vi "buildRampUpWaveform.vi"(4 "Fs":dbl=10000.0, 6 "square wave duty cycle (%)":dbl=20.0 format="%0.2f", 7 "signal type":T1(ring)=enum."Square Wave", 8 "input cluster":cluster{"Fs":dbl, "#s":dbl}={"Fs"=1000.0, "#s"=1000.0}, 9 "amplitude":dbl=2.5, 10 "freq":dbl=40.0, 11 "sec rampup":dbl=0.5 format="%#_13g") -> (3 "rampUp out":waveform(dbl)={"t0"=timestamp(0 s since 1904-01-01), "dt"=1.0, "Y"=array[62500 elements]})   [LabVIEW 2018]
uses:
  <vilib>/Waveform/WDTOps.llb/WDT Append Waveforms DBL.vi
  <vilib>/measure/NI_MABase.lvlib
panel:
  out "output cluster":cluster{"Fs":dbl, "#s":dbl}
  out "N":i32
  out "Waveform Graph":waveform(dbl)(graph)={"t0"=timestamp(0 s since 1904-01-01), "dt"=1.0, "Y"=[]} caption="Optostim waveform"
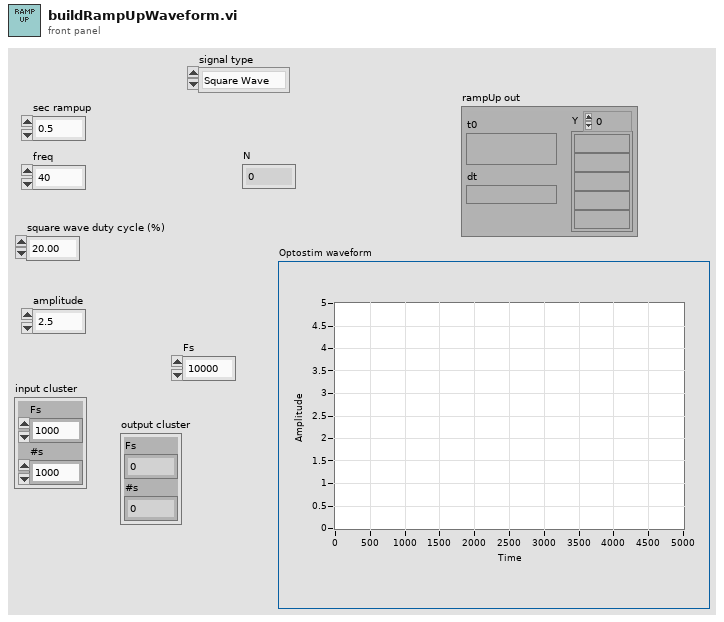
[diagram p1: front panel]
types:
  T1 = enum16{"Sine Wave", "Triangle Wave", "Square Wave", "Sawtooth Wave"}
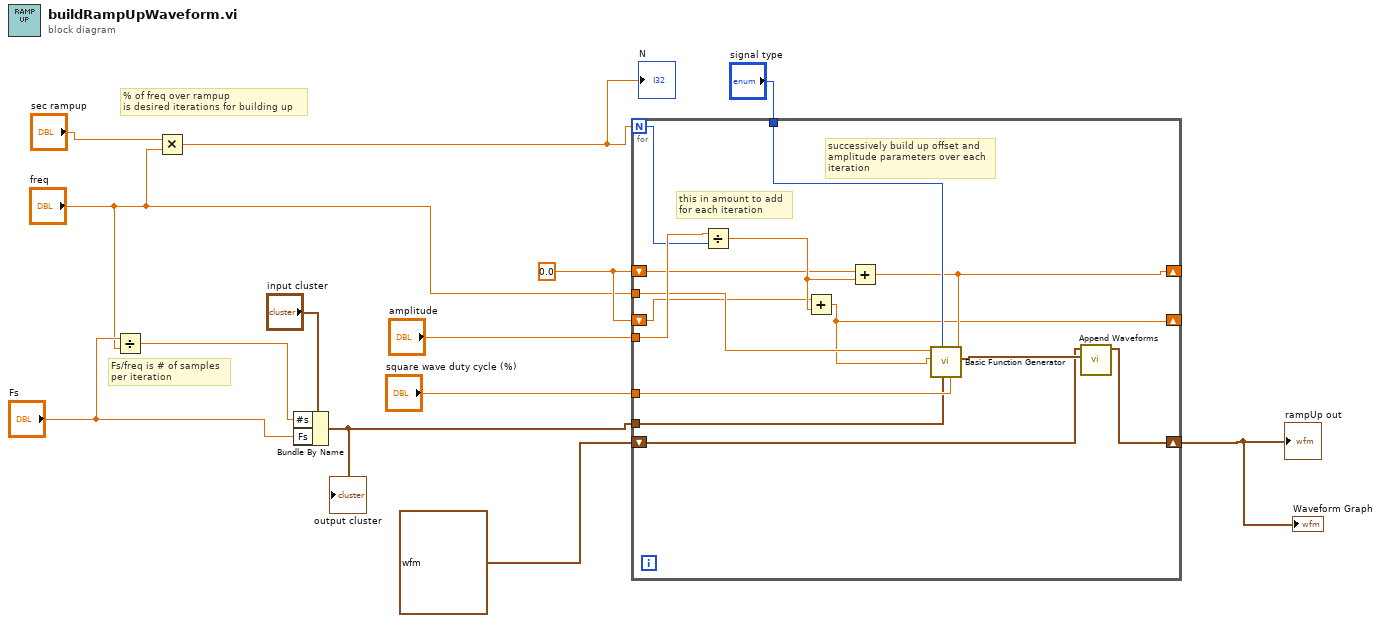
[diagram p0: block diagram]
diagram:
  w9 = 0.0
  # "% of freq over rampup \nis desired iterations for building up"
  # "Fs/freq is # of samples \nper iteration"
  n1 = Divide(x="Fs", y="freq") -> (x/y=w7:dbl)
  n2 = Multiply(x="sec rampup", y="freq") -> (x*y=w1:dbl)
  "N" <- w1
  n3 = Bundle By Name(cluster="input cluster", "#s"=w7, "Fs"="Fs") -> (w6:cluster{"Fs":dbl, "#s":dbl})
  "output cluster" <- w6
  n4 = for {
    N: w1 -> [w22]
    shift-right: [w24] -> w3
    shift-left: waveform(dbl) {"t0"=timestamp(0 s since 1904-01-01), "dt"=1.0, "Y"=[]} ("signal out") -> [w25]
    tunnel: "amplitude" -> [w23]
    shift-right: [w17] -> _
    shift-left: w9 -> [w18]
    tunnel: "signal type" -> [w21]
    tunnel: "freq" -> [w20]
    tunnel: "square wave duty cycle (%)" -> [w19]
    shift-right: [w16] -> _
    shift-left: w9 -> [w15]
    tunnel: w6 -> [w14]
    # "this in amount to add\nfor each iteration"
    # "successively build up offset and \namplitude parameters over each\niteration"
    n5 = Divide(x=w23, y=w22) -> (x/y=w27:dbl)
    n6 = Add(x=w15, y=w27) -> (x+y=w16:dbl)
    n7 = Add(x=w18, y=w27) -> (x+y=w17:dbl)
    n8 = call <vilib>:"Basic Function Generator.vi"("offset"=w17, "square wave duty cycle (%)"=w19, "sampling info"=w14, "signal type"=w21, "amplitude"=w16, "frequency"=w20) -> ("signal out"=w26:waveform(dbl))  [unwired: 3 in, 2 out]
    n9 = call-poly <vilib>:"Append Waveforms.vi"("waveform B"=w26, "waveform A"=w25) -> ("waveform out"=w24:waveform(dbl))  [unwired: 8 in, 1 out]
  }
  "rampUp out" <- w3
  "Waveform Graph" <- w3
